vi "PhaseShifter demo run init.vi"(7 "VNA ports":bool[](array[boolean])=[FALSE, FALSE, TRUE, TRUE], 9 "De-embedding files in":path[](array[path]), 10 "Toggle 6.lvclass in":refnum<class "Toggle 6.lvclass">, 11 "Vector Network Analyzer.lvclass in":refnum<class "Vector Network Analyzer.lvclass">) -> (1 "De-embedding files":path[](array[path]), 2 "Toggle 6.lvclass":refnum<class "Toggle 6.lvclass">, 3 "Vector Network Analyzer.lvclass":refnum<class "Vector Network Analyzer.lvclass">)   [LabVIEW 2020]
uses:
  Instruments/Vector Network Analyzer/Vector Network Analyzer.lvclass
  Devices/Toggle 6/Toggle 6.lvclass
  Instruments/Vector Network Analyzer/Controls/S parm format enum.ctl
  Devices/Toggle 6/Controls/Test Sequence.ctl
  Devices/Controls/Register to Write.ctl
  Devices/Toggle 6/Controls/EFuse modes enum.ctl
  <vilib>/addons/HF Network Analysis/Support VIs/Read SnP File (SnP).vi
  <vilib>/addons/HF Network Analysis/NI_HFNetworkAnalysis.lvlib
  Devices/PIC-device/PIC-Device.lvclass
panel:
  in  "S parameter":T1(ring)
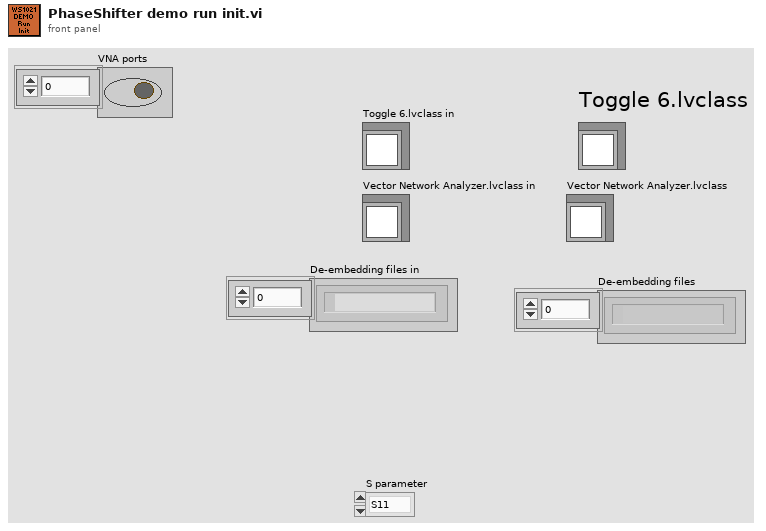
[diagram p1: front panel]
types:
  T1 = enum16{"S11", "S21", "S31", "S41", "S22", "S12", "S32", "S42", "S33", "S13", "S23", "S43", "S44", "S14", "S24", "S34"}
  T2 = typedef "Toggle 6.lvclass/Test Sequence.ctl" = cluster{"Charge Pump Settings":T3[], "Charge Pump Values":dbl[], "Efuse Register Array":T3[], "Efuse Array":T4[], "Cap Register Array":T3[], "Cap Value Array":cluster{"Register Number":u32, "Value":dbl}[]}
  T3 = typedef "PIC-Device.lvclass/Register to Write.ctl" = cluster{"Register":u32, "Value":u32, "Dev Address":u32, "Physical Adress":u32}
  T4 = typedef "Toggle 6.lvclass/EFuse modes enum.ctl" = enum16{"On", "Off", "Both On and Off"}
  T5 = typedef "Vector Network Analyzer.lvclass/S parm format enum.ctl" = enum16{"Mag dB", "Mag", "Phase", "Smith", "Real", "Imag", "Group Delay", "SWR"}
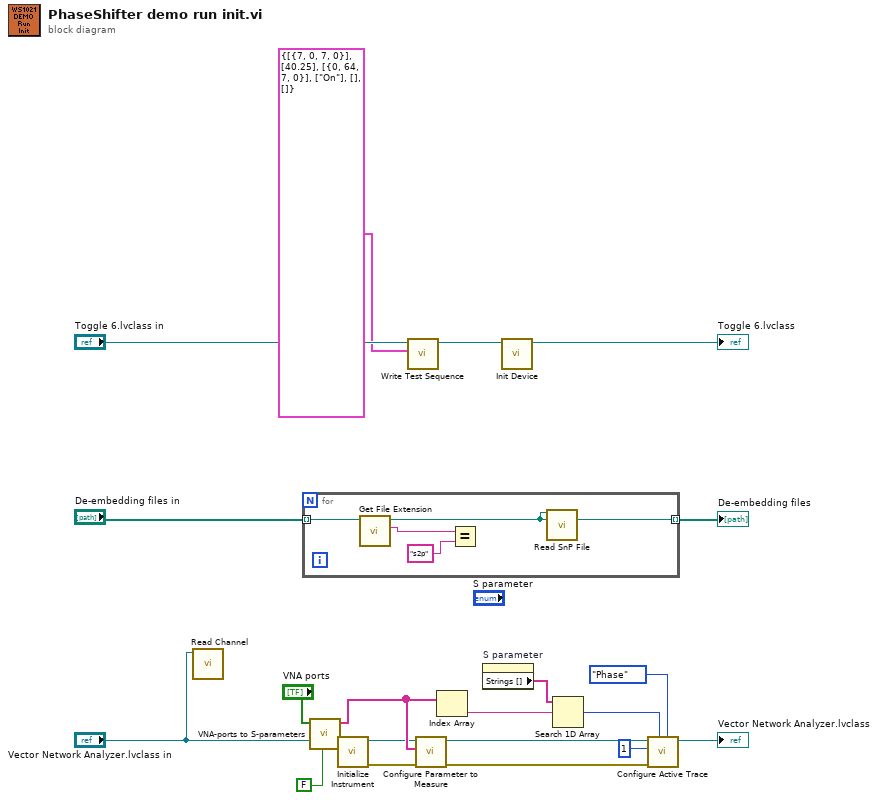
[diagram p0: block diagram]
diagram:
  n1 = call-dynamic "Read Channel.vi"("Vector Network Analyzer in"="Vector Network Analyzer.lvclass in") -> ()  [unwired: 9 in, 2 out]
  n2 = for {
    tunnel: "De-embedding files in" -> [w24] mode=indexing
    tunnel: [w21] -> w18 mode=indexing
    n3 = call <vilib>:"Get File Extension.vi"("file"=w24) -> ("lowercase file extension"=w23:string, "dup file"=w21:path)  [unwired: 6 in, 3 out]
    n4 = Equal?(x=w23, y="s2p" ("lowercase file extension")) -> ()  [unwired: 1 out]
    n5 = call-poly <vilib>:"Read SnP File.vi"("SnP File Path"=w21) -> ()  [unwired: 11 in, 4 out]
  }
  "De-embedding files" <- w18
  n6 = call "VNA-ports to S-parameters.vi"("VNA ports"="VNA ports") -> ("Sparameters (string)"=w9:string[])  [unwired: 6 in, 4 out]
  n7 = call-dynamic "Initialize Instrument.vi"("Reset"=FALSE, "Instrument in"="Vector Network Analyzer.lvclass in") -> ("error out"=w5:errorcluster, "Instrument out"=w7:refnum<class "Vector Network Analyzer.lvclass">)  [unwired: 8 in]
  n8 = call-dynamic "Write Test Sequence.vi"("Test Sequence"=T2 {"Charge Pump Settings"=[{"Register"=7, "Value"=0, "Dev Address"=7, "Physical Adress"=0}], "Charge Pump Values"=[40.25], "Efuse Register Array"=[{"Register"=0, "Value"=64, "Dev Address"=7, "Physical Adress"=0}], "Efuse Array"=[enum."On"], "Cap Register Array"=[], "Cap Value Array"=[]} ("Test Sequence 2"), "Toggle 6 in"="Toggle 6.lvclass in") -> ("Toggle 6 out"=w3:refnum<class "Toggle 6.lvclass">)  [unwired: 9 in]
  n9 = call-dynamic "Configure Parameter to Measure.vi"("error in (no error)"=w5, "Sparameters (string)"=w9, "Vector Network Analyzer in"=w7) -> ("error out"=w16:errorcluster, "Vector Network Analyzer out"=w15:refnum<class "Vector Network Analyzer.lvclass">)  [unwired: 7 in]
  n10 = Index Array(array=w9) -> (element=w11:string)  [unwired: 1 in]
  n11 = property on="S parameter" class="Enum (strict)"() -> ("Strings []"=w12:string[])  [unwired: 2 in, 2 out]
  n12 = call-dynamic "Init Device.vi"("Toggle 6 in"=w3) -> ("Toggle 6 out"=→"Toggle 6.lvclass":refnum<class "Toggle 6.lvclass">)  [unwired: 9 in, 1 out]
  n13 = Search 1D Array(1D array=w12, element=w11) -> (index of element=w10:i32)  [unwired: 1 in]
  n14 = call-dynamic "Configure Active Trace.vi"("Format"=S_parm_format_enum."Phase", "S parameter"=w10, "error in (no error)"=w16, "Active Trace"=u8 1, "Vector Network Analyzer in"=w15) -> ("Vector Network Analyzer out"=→"Vector Network Analyzer.lvclass":refnum<class "Vector Network Analyzer.lvclass">)  [unwired: 5 in, 1 out]
